vi "example1.vi"(9 "Discesa":dbl[][](array[numeric])) -> (0 "incertezza_comb":dbl[](array[numeric]), 1 "incertezza discesa":dbl, 2 "incertezza_composta":dbl, 3 "incertezza salita":dbl, 4 "u_a22":dbl[](array[numeric]), 5 "u_a12":dbl[](array[numeric]), 6 "ari_mean discesa":dbl[](array[numeric]), 7 "ari_mean salita":dbl[](array[numeric]))   [LabVIEW 2021]
uses:
  CALIBRATION.lvlib
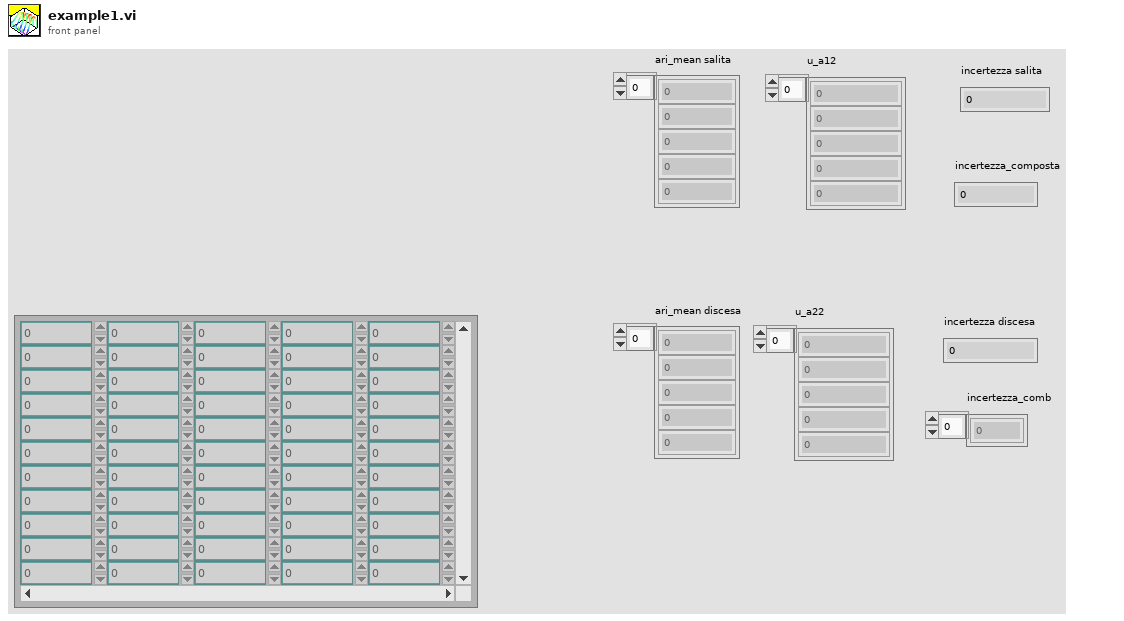
[diagram p1: front panel]
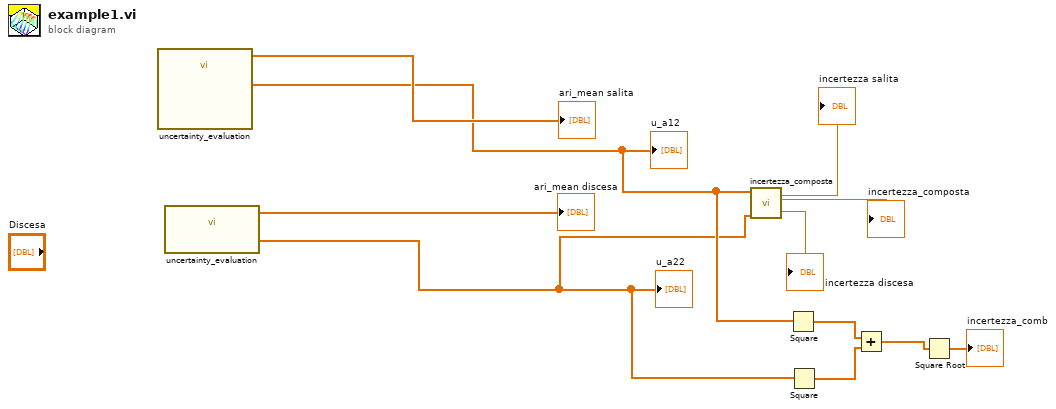
[diagram p0: block diagram]
diagram:
  n1 = call "uncertainty_evaluation.vi"() -> ("combined_uncertainty"=w6:dbl[], "expected_value"=→"ari_mean salita":dbl[])  [unwired: 3 in]
  "u_a12" <- w6
  n2 = call "uncertainty_evaluation.vi"() -> ("combined_uncertainty"=w5:dbl[], "expected_value"=→"ari_mean discesa":dbl[])  [unwired: 3 in]
  "u_a22" <- w5
  n3 = call "incertezza_composta.vi"("Descending uncertainty point-by-point"=w5, "Ascending uncertainty point-by-point"=w6) -> ("incertezza_composta"=→"incertezza_composta":dbl, "ascending_uncertainty (absolute value)"=→"incertezza discesa":dbl, "descending_uncertainty (absolute value)"=→"incertezza salita":dbl)  [unwired: 7 in]
  n4 = Square(x=w6) -> (x^2=w4:dbl[])
  n5 = Square(x=w5) -> (x^2=w3:dbl[])
  n6 = Add(x=w4, y=w3) -> (x+y=w2:dbl[])
  n7 = Square Root(x=w2) -> (sqrt(x)=→"incertezza_comb":dbl[])
